vi "New Gesture.vi"(8 "offset":T1, 9 "point":T1, 10 "elapsed time":u32, 11 "gesture":T2) -> (3 "gesture out":refnum<class "Gesture.lvclass">)   [LabVIEW 2019, in "Gesture.lvclass"]
doc: "Create a new Gesture object."
uses:
  Gesture.lvclass
  Gesture Enum.ctl
  <vilib>/Utility/miscctls.llb/LVPoint32TypeDef.ctl
  Gesture.lvclass/Gesture.ctl
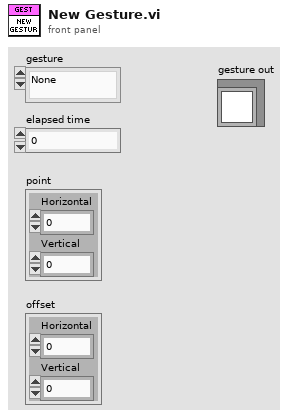
[diagram p1: front panel]
types:
  T1 = typedef "LVPoint32TypeDef.ctl" = cluster{"Horizontal":i32, "Vertical":i32}
  T2 = typedef "Gesture.lvclass/Gesture Enum.ctl" = enum16{"None", "Stop", "Tap", "Press", "Pan Start", "Pan Continue", "Pan End", "Pinch Open", "Pinch Close", "Double Tap"}
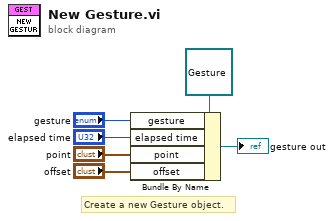
[diagram p0: block diagram]
diagram:
  # "Create a new Gesture object."
  n1 = Bundle By Name(cluster=refnum<class "Gesture.lvclass"> refnum ("Gesture Message"), "gesture"="gesture", "elapsed time"="elapsed time", "point"="point", "offset"="offset") -> (→"gesture out":refnum<class "Gesture.lvclass">)
